vi "Incrementer.vi"(1 "N":i32, 7 "reset":bool) -> (8 "Count":i32)   [LabVIEW 2013]
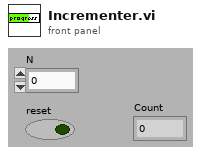
[diagram p1: front panel]
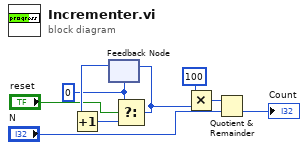
[diagram p0: block diagram]
diagram:
  w7 = 0
  n1 = feedback #1(w7) -> (w9:i32)
  n2 = Increment(x=w9) -> (x+1=w6:i32)
  n3 = Select(t=w7, s="reset", f=w6) -> (s? t:f=w2:i32)
  n4 = feedback-in #1(w2) -> ()
  n5 = Multiply(x=100, y=w2) -> (x*y=w5:i32)
  n6 = Quotient & Remainder(x=w5, y="N") -> (floor(x/y)=→"Count":i32)  [unwired: 1 out]
